vi "ExSubSetupCamPulser.vi"(3 "error in (no error)":errorcluster, 4 "Pulser data in":T1 {"Pulse Delay" format="%.2f"; "Pulse Width" format="%.2f"; "Freq" format="%.2f"}, 5 "Pulser Handle":u32, 6 "Camera Handle":u32) -> (0 "error out":errorcluster, 1 "Pulser Handle":u32, 2 "Camera Handle":u32)   [LabVIEW 2010]
panel:
  # "ExSubSetupCamPulser:\nThis Sub VI sets up the PTG as internal\ntriggering, and sets the parameters \nassociated with it, including on chip \naccumulation."
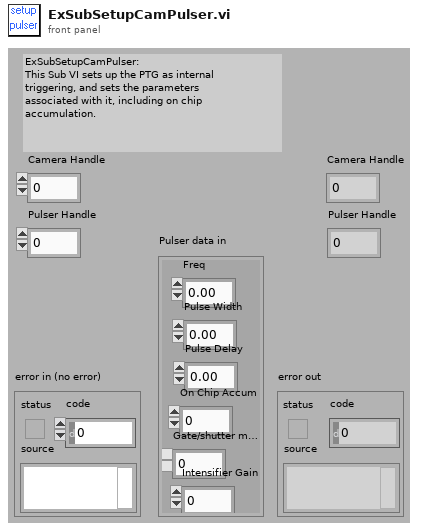
[diagram p1: front panel]
types:
  T1 = cluster{"Freq":dbl, "Pulse Width":dbl, "Pulse Delay":dbl, "On Chip Accum":u32, "Gate/shutter mode":u32, "Intensifier Gain":u32}
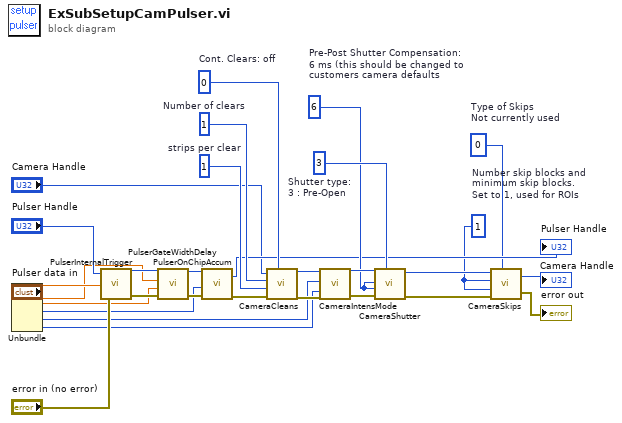
[diagram p0: block diagram]
diagram:
  w1 = 0  # Type of Skips Not currently used
  w2 = 1  # Number skip blocks and minimum skip blocks. Set to 1, used for ROIs
  w18 = 6  # Pre-Post Shutter Compensation: 6 ms (this should be changed to customers camera defaults
  w19 = 3  # Shutter type: 3 : Pre-Open
  w24 = 0  # Cont. Clears: off
  w26 = 1  # Number of clears
  w27 = 1  # strips per clear
  n1 = Unbundle("Pulser data in") -> ("Freq"=w15:dbl, "Pulse Width"=w11:dbl, "Pulse Delay"=w10:dbl, "On Chip Accum"=w9:u32, "Gate/shutter mode"=w7:u32, "Intensifier Gain"=w8:u32)
  n2 = call <userlib>:"PulserInternalTrigger.vi"("error in (no error)"="error in (no error)", "Freq"=w15, "Pulser Handle"="Pulser Handle") -> ("error out"=w31:errorcluster, "Pulser Handle"=w30:u32)
  n3 = call <userlib>:"PulserGateWidthDelay.vi"("error in (no error)"=w31, "Gate Delay"=w10, "Gate Width"=w11, "Pulser Handle"=w30) -> ("error out"=w29:errorcluster, "Pulser Handle"=w28:u32)
  n4 = call <userlib>:"PulserOnChipAccum.vi"("error in (no error)"=w29, "Accumulation"=w9, "Pulser Handle"=w28) -> ("error out"=w25:errorcluster, "Pulser Handle"=→"Pulser Handle":u32)
  n5 = call <userlib>:"CameraCleans.vi"("Camera Handle"="Camera Handle", "Number of Clears"=w26, "Number of Strips Per Clear"=w27, "error in"=w25, "Continuous Clears"=w24) -> ("Camera Handle"=w22:u32, "error out"=w23:errorcluster)
  n6 = call <userlib>:"CameraIntensMode.vi"("error in"=w23, "Intensifier Gain"=w8, "Mode"=w7, "Camera Handle"=w22) -> ("error out"=w20:errorcluster, "Camera Handle"=w21:u32)
  n7 = call <userlib>:"CameraShutter.vi"("Camera Handle"=w21, "Shutter Comp Time: Pre Open"=w18, "Shutter Comp Time: Post Open"=w18, "error in"=w20, "Shutter State"=w19) -> ("Camera Handle"=w6:u32, "error out"=w5:errorcluster)
  n8 = call <userlib>:"CameraSkips.vi"("Camera Handle"=w6, "Minimum Block Size"=w2, "Number of Minimum blocks"=w2, "error in"=w5, "Type of Skips"=w1) -> ("Camera Handle"=→"Camera Handle":u32, "error out"=→"error out":errorcluster)
